vi "DeleteRows.vi"(0 "Col Array Ref in":refnum<vi>, 1 "Start Row":i32, 2 "Layout Ring Refnum":refnum<vi>, 3 "Mode Col Index":i32, 4 "Table CtlRef In":refnum<vi>, 5 "error in (no error)":errorcluster, 6 "Table History ref":refnum<vi>, 11 "# rows":i32) -> (14 "Col Array Ref out":refnum<vi>, 18 "Table CtlRef Out":refnum<vi>, 19 "error out":errorcluster)   [LabVIEW 2013]
doc: "Delete requested row(s), properly adjusting table formatting, and renumbering rows; also saves Table History for undo/redo. While it is assumed that \"# rows\" and \"Start Row\" are in bounds, this VI won't let the user empty the SetList table (leaves 1st row)."
uses:
  TypeDefs/TableHistory.ctl
  TypeDefs/TableArray.ctl
  <vilib>/Utility/miscctls.llb/LVRowAndColumnTypeDef.ctl
  ColumnVIs/Column/Column.lvclass
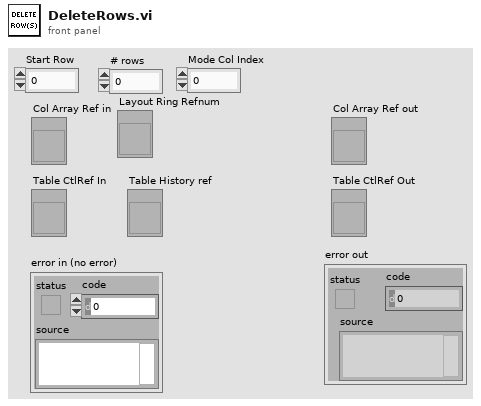
[diagram p1: front panel]
types:
  T1 = typedef "LVRowAndColumnTypeDef.ctl" = cluster{"Row":i32, "Column":i32}
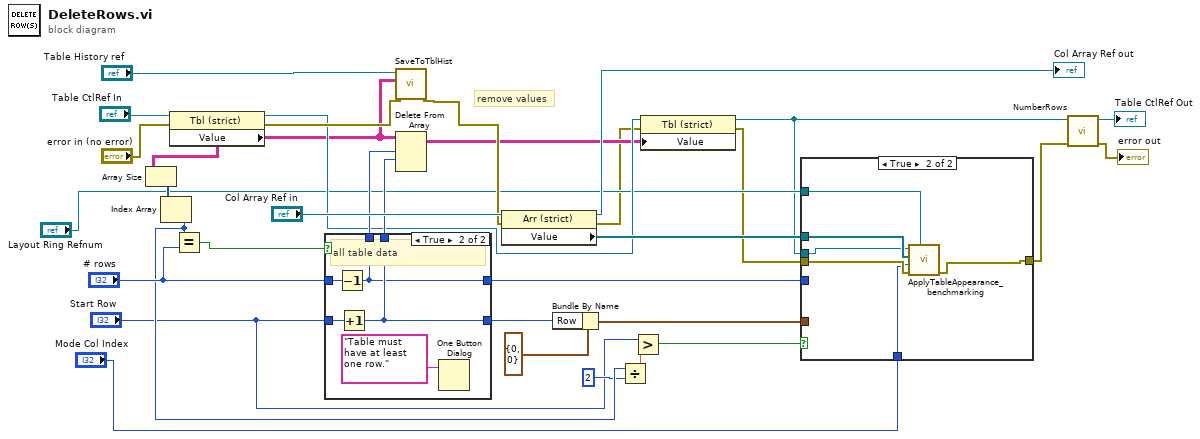
[diagram p0: block diagram]
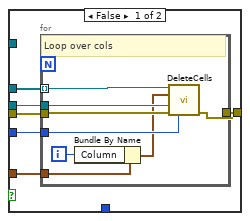
[diagram p2: hidden frame]
diagram:
  # "remove values"
  n1 = property class="Tbl (strict)"(reference="Table CtlRef In", error in="error in (no error)") -> (reference out=w15:refnum<vi>, error out=w26:errorcluster, "Value"=w14:string[][])
  n2 = Array Size(array=w14) -> (size(s)=w25:i32[])
  n3 = Index Array(array=w25) -> (element=w10:i32)  [unwired: 1 in]
  n4 = Equal?(x=w10, y="# rows") -> (x = y?=w23:bool)
  n5 = case shown="True" w23 {
    tunnel: "# rows" -> [w35 w40]
    tunnel: "Start Row" -> [w34 w39]
    tunnel: [w34 w38] -> w24
    tunnel: [w34 w38] -> w21
    tunnel: [w35 w36] -> w22
    tunnel: [w35 w36] -> w20
    frame False {
      # "not entire table data"
    }
    frame True {
      # "all table data"
      n6 = Decrement(x=w40) -> (x-1=w36:i32)
      n7 = Increment(x=w39) -> (x+1=w38:i32)
      n8 = One Button Dialog(message="Table must have at least one row.") -> ()  [unwired: 1 in, 1 out]
    }
  }
  n9 = call "SaveToTblHist.vi"("error in (no error)"=w26, "OldTable (reset)"=w14, "Table History ref"="Table History ref") -> ("error out"=w16:errorcluster)  [unwired: 8 in]
  n10 = Delete From Array "Delete From Array"(array=w14, length=w20, index (row)=w21) -> (array with subset deleted=w13:string[][])  [unwired: 1 in, 1 out]
  n11 = property class="Arr (strict)"(reference="Col Array Ref in", error in=w16) -> (reference out=→"Col Array Ref out":refnum<vi>, error out=w5:errorcluster, "Value"=w30:refnum<class "Column.lvclass">[])
  n12 = Bundle By Name(cluster=T1 {"Row"=0, "Column"=0} ("Active Cell:Active Cell"), "Row"=w24) -> (w28:T1)
  n13 = Divide(x=w10, y=2) -> (x/y=w11:dbl)
  n14 = Greater?(x="Start Row", y=w11) -> (0:w2:bool)
  n15 = property class="Tbl (strict)"(reference=w15, error in=w5, "Value"=w13) -> (reference out=w6:refnum<vi>, error out=w4:errorcluster)
  n16 = case shown="True" w2 {
    tunnel: [w46 w60] -> w3
    tunnel: w30 -> [w45 w58]
    tunnel: w4 -> [w44 w59]
    tunnel: w28 -> [w43 _]
    tunnel: w22 -> [w42 _]
    tunnel: w6 -> [w41 w57]
    tunnel: "Layout Ring Refnum" -> [_ w56]
    tunnel: "Mode Col Index" -> [_ w55]
    frame False {
      n17 = for {
        tunnel: w44 -> [w53]
        tunnel: [w47] -> w46
        tunnel: w45 -> [w51] mode=indexing
        tunnel: w42 -> [w50]
        tunnel: w43 -> [w49]
        tunnel: w41 -> [w52]
        i -> [w54]
        # "Loop over cols"
        n18 = Bundle By Name(cluster=w49, "Column"=w54) -> (w48:T1)
        n19 = call-dynamic "DeleteCells.vi"("Column in"=w51, "Cell Position"=w48, "Table CtlRef In"=w52, "error in (no error)"=w53, "# Rows"=w50) -> ("error out"=w47:errorcluster)  [unwired: 8 in, 2 out]
      }
    }
    frame True {
      n20 = call "ApplyTableAppearance_benchmarking.vi"("Layout Ring Ref"=w56, "error in (no error)"=w59, "Mode Index"=w55, "Col Array in"=w58, "Table Ref in"=w57) -> ("error out"=w60:errorcluster)  [unwired: 5 in, 1 out]
    }
  }
  n21 = call "NumberRows.vi"("error in (no error)"=w3, "Table Ref in"=w6) -> ("error out"=→"error out":errorcluster, "Table Ref out"=→"Table CtlRef Out":refnum<vi>)  [unwired: 8 in]
